vi "SetExternalTransferFunction.vi"(0 "Ext. Transfer Funct. Cluster":T1={"Number"=0, "Offset"=-inf, "Gain [Unit/V]"=-inf, "Unit"=-2147483648} {"Unit" items=["[read only]"=-2147483648, "Not Valid"=128, "m"=384, "mm"=383, "um"=382, "nm"=381, "pm"=380, "V"=640, "mV"=639, "uV"=638, "nV"=637, "MHz"=898, "kHz"=897, "Hz"=896, "mHz"=895, "Ks"=1153, "s"=1152, "ms"=1151, "us"=1150, "ns"=1149, "ps"=1148, "A"=1408, "mA"=1407, "uA"=1406, "nA"=1405, "W"=1664, "mW"=1663, "uW"=1662, "nW"=1661, "T"=1920, "mT"=1919, "uT"=1918, "nT"=1917, "K"=2176, "mK"=2175, "uK"=2174, "nK"=2173, "Deg"=2432, "mDeg"=2431, "uDeg"=2430, "nDeg"=2429, "[cos]"=2688, "[dB]"=2944, "LSB"=3200]; "Offset" format="%#_g mV"; "Number" items=["ADC 1", "ADC 2", "ADC 3", "ADC 4", "ADC 5", "ADC 6"]}, 5 "error in":T4) -> (14 "Output Cluster":T1={"Number"=0, "Offset"=-inf, "Gain [Unit/V]"=-inf, "Unit"=-2147483648} {"Unit" items=["[read only]"=-2147483648, "Not Valid"=128, "m"=384, "mm"=383, "um"=382, "nm"=381, "pm"=380, "V"=640, "mV"=639, "uV"=638, "nV"=637, "MHz"=898, "kHz"=897, "Hz"=896, "mHz"=895, "Ks"=1153, "s"=1152, "ms"=1151, "us"=1150, "ns"=1149, "ps"=1148, "A"=1408, "mA"=1407, "uA"=1406, "nA"=1405, "W"=1664, "mW"=1663, "uW"=1662, "nW"=1661, "T"=1920, "mT"=1919, "uT"=1918, "nT"=1917, "K"=2176, "mK"=2175, "uK"=2174, "nK"=2173, "Deg"=2432, "mDeg"=2431, "uDeg"=2430, "nDeg"=2429, "[cos]"=2688, "[dB]"=2944, "LSB"=3200]; "Offset" format="%#_g mV"; "Number" items=["ADC 1", "ADC 2", "ADC 3", "ADC 4", "ADC 5", "ADC 6"]}, 19 "error out":T4)   [LabVIEW 2016]
doc: "This VI sets up an external transfer function. The input cluster contains the following parameters.\n- Number (integer) [0 to 2]\n- Gain in Unit per volt (float) [without restraint]\n- Offset in mV (float) [without restraint]\n- Unit (integer) [0 -- mm; 1 -- um; 2 -- nm; 3 -- pm; 4 -- V; 5 -- mV; 6 -- uV; 7 -- nV; 8 -- MHz; 9 -- kHz; 10 -- Hz; 11 -- mHz; 12 -- s; 13 -- ms; 14 -- us; 15 -- ns; 16 -- A; 17 -- mA; 18 -- uA; 19 -- nA; 20 -- [cos]; 24 -- [dB]; 32 -- W; 33 -- mW; 34 -- uW; 35 -- nW]\nBy passing -Inf (float) or -2147483648 (integer) as input values, the corresponding parameter(s) will be read out."
uses:
  Controls/External-Transfer-Function_Parameters.ctl
  Controls/External-Transfer-Function_Selection.ctl
  Controls/External-Transfer-Function-Unit_Selection.ctl
  Controls/Error_Out.ctl
  Files_ASC500/DLL/ASC500_RemoteControlV27.dll
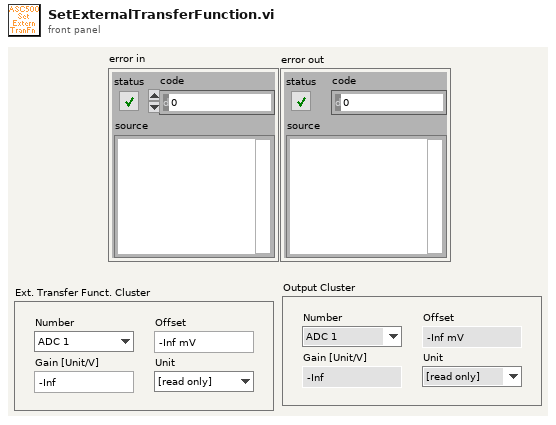
[diagram p1: front panel]
types:
  T1 = typedef "External-Transfer-Function_Parameters.ctl" = cluster{"Number":T2, "Offset":sgl, "Gain [Unit/V]":dbl, "Unit":T3}
  T2 = typedef "External-Transfer-Function_Selection.ctl" = u16
  T3 = typedef "External-Transfer-Function-Unit_Selection.ctl" = i32
  T4 = typedef "Error_Out.ctl" = errorcluster
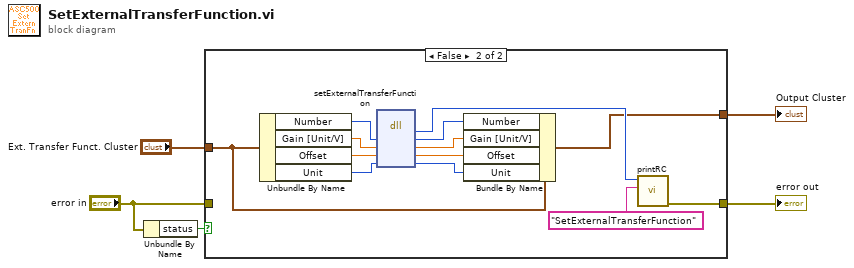
[diagram p0: block diagram]
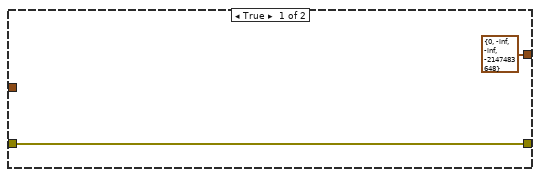
[diagram p2: hidden frame]
diagram:
  n1 = Unbundle By Name("error in") -> ("status"=w4:bool)
  n2 = case shown="False" w4 {
    tunnel: [w6 w12] -> w5
    tunnel: "Ext. Transfer Funct. Cluster" -> [_ w14]
    tunnel: [T1 {"Number"=0, "Offset"=-inf, "Gain [Unit/V]"=-inf, "Unit"=-2147483648} ("External Transfer Function Cluster") w8] -> w1
    tunnel: "error in" -> [w6 _]
    frame True {
    }
    frame False {
      n3 = Unbundle By Name(w14) -> ("Number"=w18:T2, "Gain [Unit/V]"=w19:dbl, "Offset"=w13:sgl, "Unit"=w20:T3)
      n4 = dll-call lib="G:/SCMOperations/Share/ELE/Produkt Information/ASC500/04 Remote Control/02 development versions/2018Nov06/Files_ASC500/DLL/ASC500_RemoteControlV27.dll" fn="setExternalTransferFunction"("Number"=w18, "Gain"=w19, "Offset"=w13, "Unit"=w20) -> ("return type"=w11:i32, "Number"=w15:i32, "Gain"=w16:sgl, "Offset"=w17:sgl, "Unit"=w9:i32)  [unwired: 3 in, 2 out]
      n5 = Bundle By Name(cluster=w14, "Number"=w15, "Gain [Unit/V]"=w16, "Offset"=w17, "Unit"=w9) -> (w8:T1)
      n6 = call "printRC.vi"("additional information"="SetExternalTransferFunction", "RC"=w11) -> ("error out"=w12:T4)  [unwired: 9 in]
    }
  }
  "error out" <- w5
  "Output Cluster" <- w1
